vi "Meas Proc QWTB Export Result.vi"(8 "error in":errorcluster, 10 "export data":string[][](array[string]), 11 "qwtb view":T2) -> (0 "error out":errorcluster)   [LabVIEW 2020]
doc: "QWTB result export panel."
uses:
  Meas Proc QWTB Export Mode.ctl
  MEas Proc QWTB Export Sheet Name Mode.ctl
  Meas Proc QWTB Viewer References.ctl
  Meas Proc QWTB View Max Dim.ctl
  Meas Proc QWTB View Uncertainty Mode.ctl
  Meas Proc QWTB View Group Mode.ctl
  Meas Proc QWTB View Phase Mode.ctl
  Meas Proc QWTB Export Sheet Pos.ctl
  varilib/SGUI Assign References Mode.ctl
  Excel/axex_cell_xy.ctl
  GUI/GUI Waveform Info.ctl
  <vilib>/Utility/miscctls.llb/LVRowAndColumnTypeDef.ctl
  Excel/axex_write_cells.vi
  varilib/varilib.lvlib
  Excel/AX Excel.lvlib
panel:
  in  "btn refresh":bool
  in  "sheet pos":T1 caption="New worksheet position"
  in  "trg workbook":u16(ring) caption="Target workbook" items=[">>> No Workbooks <<<"]
  in  "comment":string caption="Comment (Shift+Enter to break line)"
  in  "cb add header":bool caption="Append session header"
  in  "btn cancel":bool
  in  "btn export":bool
  out "sh name prev":string caption="Sheet name preview"
  in  "sh name mode":T3=enum."%Alg Name% %timestamp%" caption="Auto name"
  in  "sh name":string caption="New sheet name"
  in  "exp mode":T4 caption="Export mode"
  out "tbl preview":string[][](table) caption="Preview"
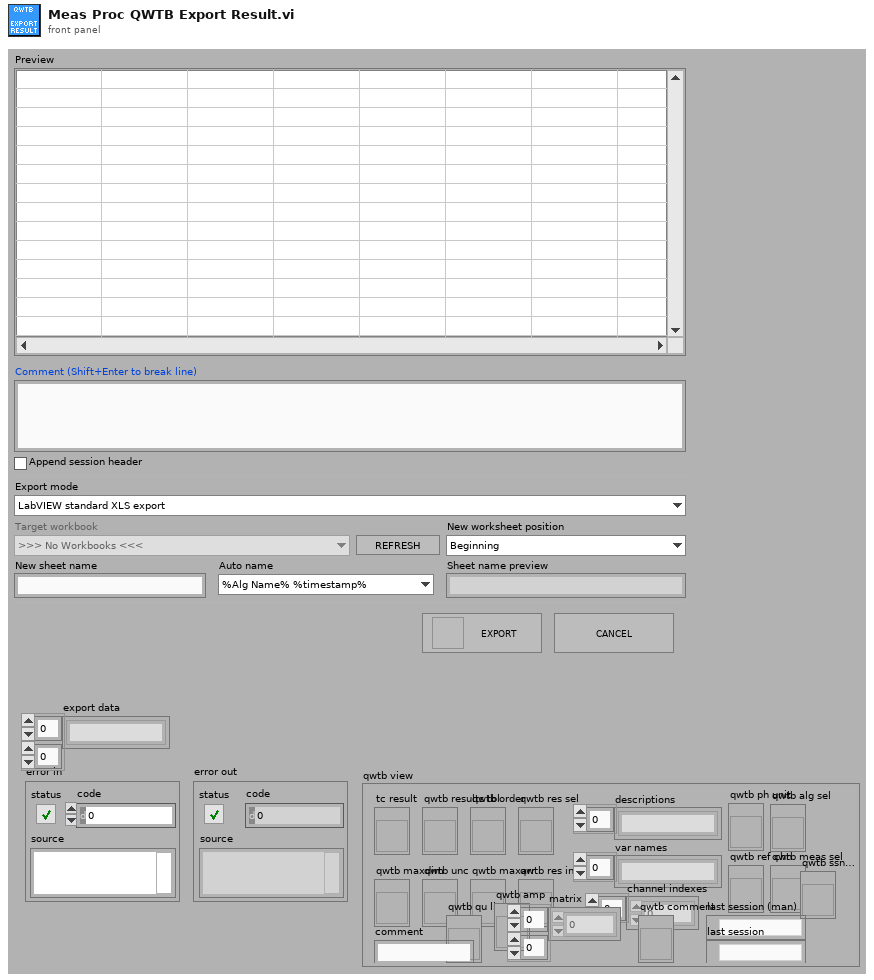
[diagram p1: front panel]
types:
  T1 = typedef "Meas Proc QWTB Export Sheet Pos.ctl" = enum16{"Beginning", "End"}
  T2 = typedef "Meas Proc QWTB Viewer References.ctl" = cluster{"tc result":refnum<vi>, "qwtb results tbl":refnum<vi>, "qwtb maxdim":refnum<vi>, "qwtb unc":refnum<vi>, "qwtb order":refnum<vi>, "qwtb maxarr":refnum<vi>, "qwtb res sel":refnum<vi>, "qwtb res info":refnum<vi>, "descriptions":string[], "var names":string[], "channel indexes":i32[], "qwtb ref chn":refnum<vi>, "qwtb ph unit":refnum<vi>, "qwtb alg sel":refnum<vi>, "qwtb meas sel":refnum<vi>, "qwtb ssn info":refnum<vi>, "last session (man)":path, "qwtb qu list":refnum<vi>, "qwtb amp":refnum<vi>, "matrix":dbl[][], "comment":string, "qwtb comment":refnum<vi>, "last session":path}
  T3 = typedef "MEas Proc QWTB Export Sheet Name Mode.ctl" = enum16{"No", "%Sheet Name% %timestamp%", "%Alg Name% %timestamp%"}
  T4 = typedef "Meas Proc QWTB Export Mode.ctl" = enum16{"LabVIEW standard XLS export", "AX Excel to active workbook", "AX Excel to selected workbook", "AX Excel to new workbook"}
  T5 = typedef "varilib.lvlib/SGUI Assign References Mode.ctl" = enum16{"Add to stack", "Overwrite", "Release last", "Release ID"}
  T6 = typedef "AX Excel.lvlib/axex_cell_xy.ctl" = cluster{"column":i32, "row":i32, "cell name":string}
  T7 = typedef "LVRowAndColumnTypeDef.ctl" = cluster{"Row":i32, "Column":i32}
  T8 = typedef "GUI Waveform Info.ctl" = cluster{"header path":path, "group id":i32, "average id":i32, "Time Stamp":timestamp, "max samples":i64, "first sample":i64, "first smpl [%]":dbl, "kill viewer":bool}
  T9 = typedef "AX Excel.lvlib/axex_instance.ctl" = cluster{"file path":path, "current sheet name":string, "sheet ref":refnum<k7>, "wbook ref":refnum<k7>}
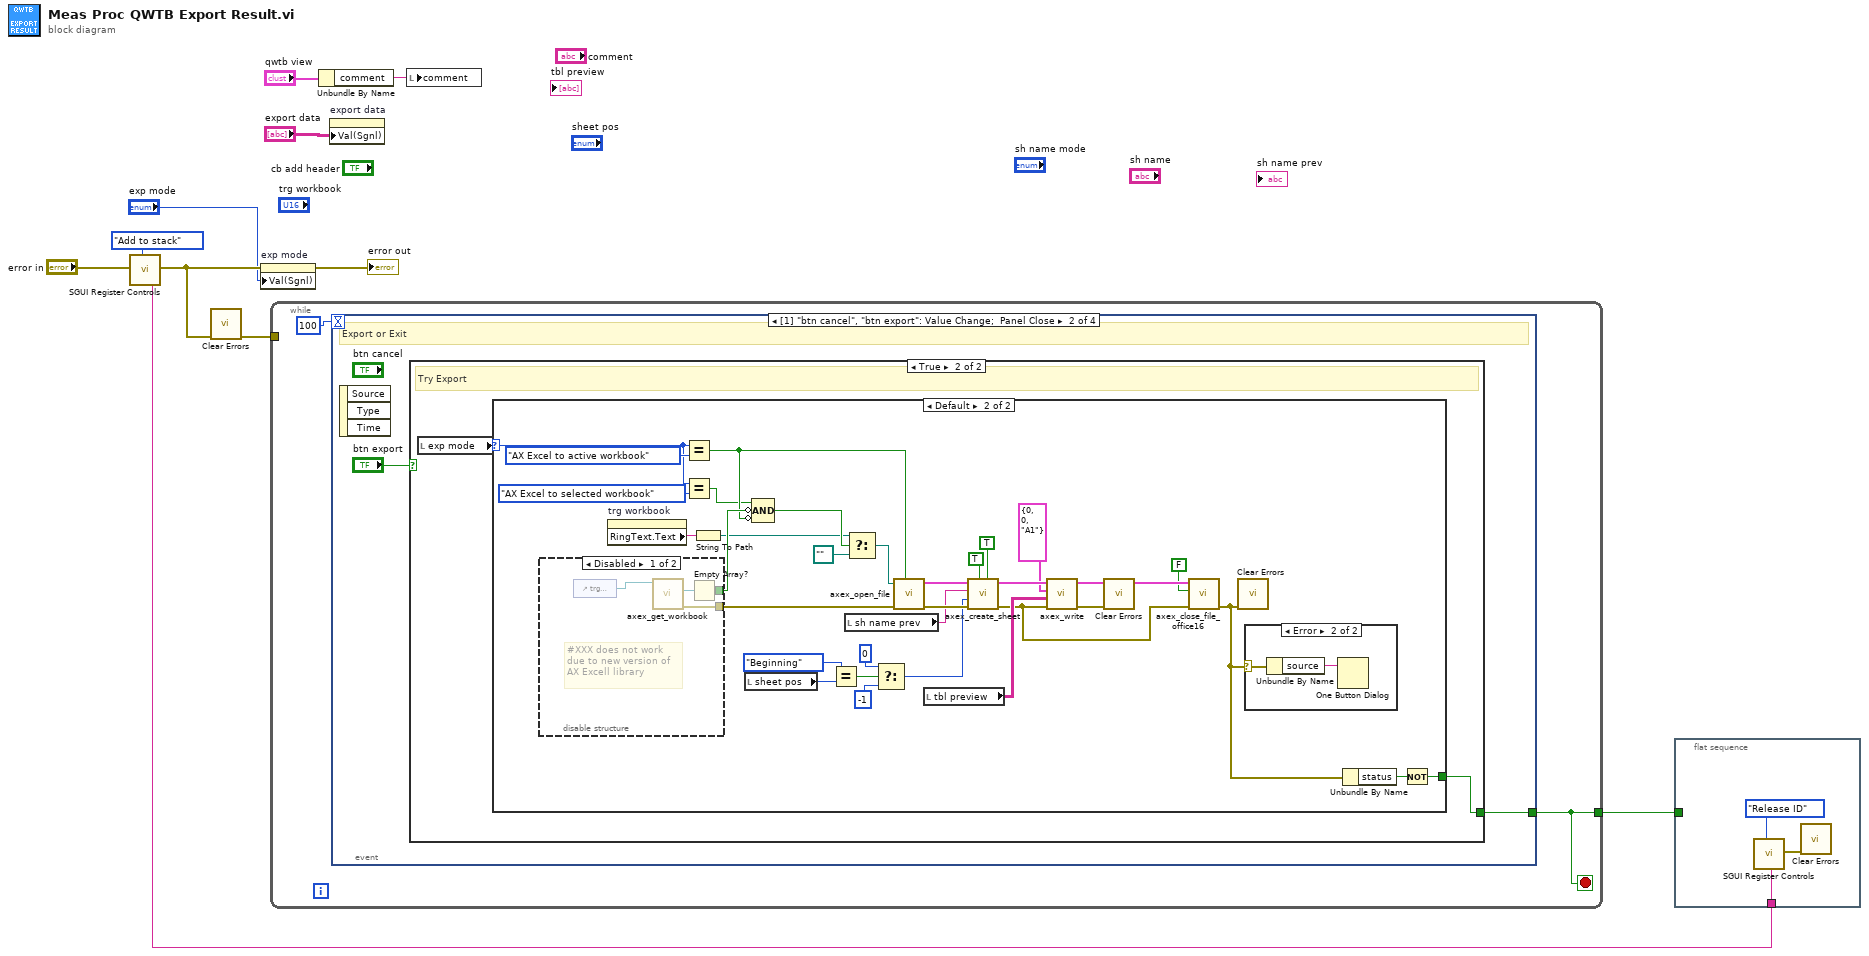
[diagram p0: block diagram]
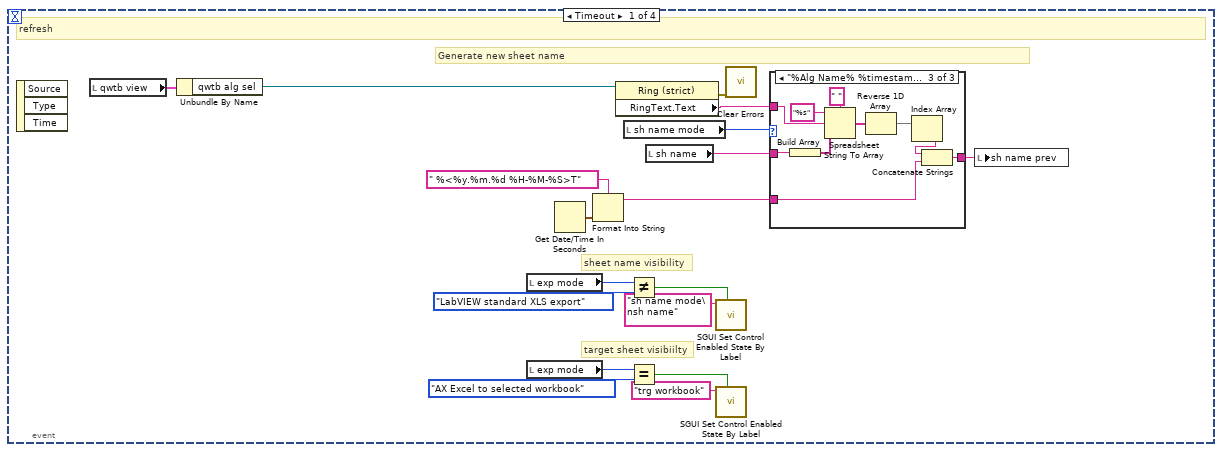
[diagram p2: hidden frame]
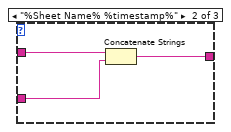
[diagram p4: hidden frame]
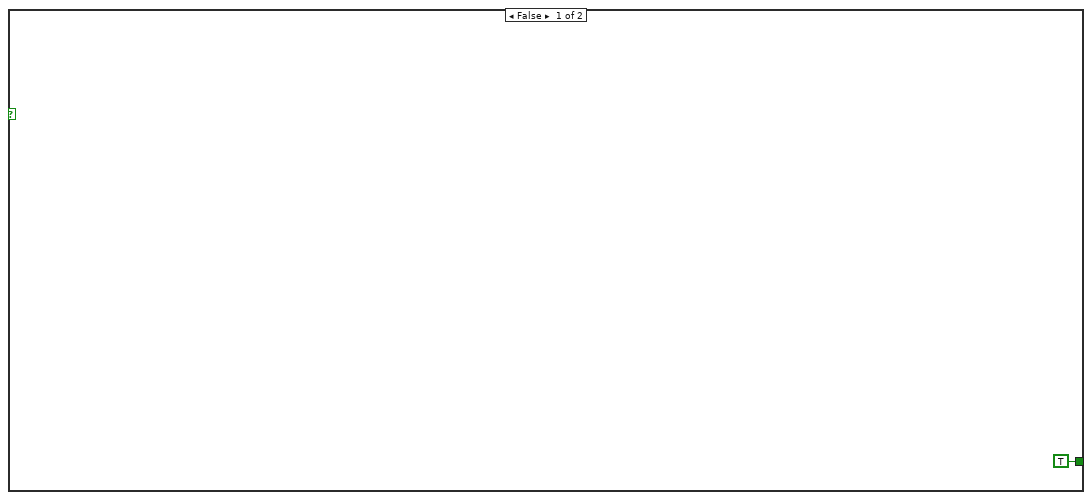
[diagram p5: hidden frame]
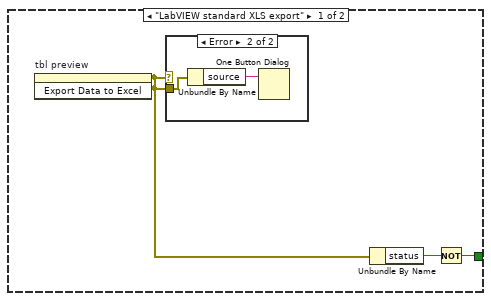
[diagram p6: hidden frame]
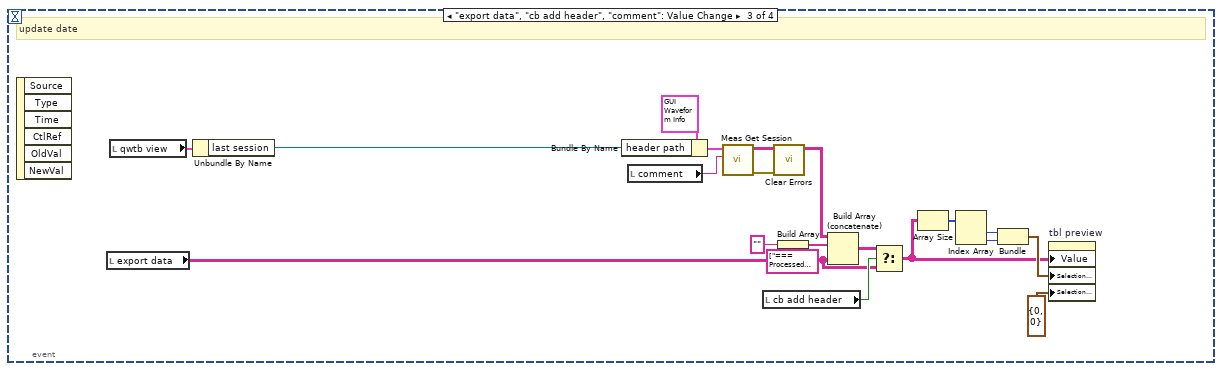
[diagram p10: hidden frame]
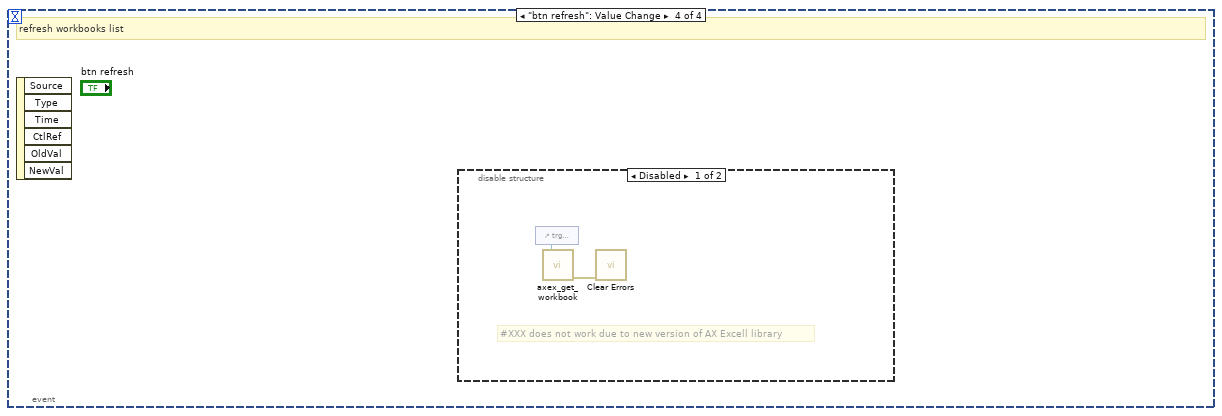
[diagram p11: hidden frame]
diagram:
  n1 = call "SGUI Register Controls.vi"("error in"="error in", "register mode (overwrite)"=SGUI_Assign_References_Mode."Add to stack") -> ("assigned ID"=w8:string, "error out"=w3:errorcluster)  [unwired: 15 in, 1 out]
  n2 = call <vilib>:"Clear Errors.vi"("error in (no error)"=w3) -> ("error out"=w9:errorcluster)  [unwired: 5 in, 1 out]
  n3 = property on="exp mode" class="Enum (strict)"(error in=w3, "Val(Sgnl)"="exp mode") -> (error out=→"error out":errorcluster)  [unwired: 1 in, 1 out]
  n4 = while {
    tunnel: w9 -> [_]
    tunnel: [w13] -> w7
    stop <- w13 stop-if-true
    n5 = event shown="[1] \"btn cancel\", \"btn export\": Value Change;  Panel Close" {
      selector: _ -> [_ _ _ _]
      dyn-events: _ -> [_ _ _ _]
      timeout: 100 -> [_ _ _ _]
      tunnel: [_ w46 _ _] -> w13
      event Timeout {
        # "target sheet visibiilty"
        # "sheet name visibility"
        # "Generate new sheet name"
        # "refresh"
        n6 = event-data() -> ()  [unwired: 1 in, 3 out]
        n7 = local read "qwtb view"() -> (w31:T2)
        n8 = Unbundle By Name(w31) -> ("qwtb alg sel"=w30:refnum<vi>)
        n9 = local read "exp mode"() -> (w22:T4)
        n10 = local read "exp mode"() -> (w14:T4)
        n11 = Get Date/Time In Seconds() -> (seconds since 1Jan1904=w25:timestamp)
        n12 = Format Into String(format string=" %<%y.%m.%d %H-%M-%S>T", w25) -> (resulting string=w24:string)  [unwired: 2 in, 1 out]
        n13 = property class="Ring (strict)"(reference=w30) -> (error out=w18:errorcluster, "RingText.Text"=w27:string)  [unwired: 1 in, 1 out]
        n14 = local read "sh name mode"() -> (w29:T3)
        n15 = Not Equal?(x=w22, y=Meas_Proc_QWTB_Export_Mode."LabVIEW standard XLS export") -> (x != y?=w20:bool)
        n16 = Equal?(x=w14, y=Meas_Proc_QWTB_Export_Mode."AX Excel to selected workbook") -> (x = y?=w16:bool)
        n17 = local read "sh name"() -> (w28:string)
        n18 = call "SGUI Set Control Enabled State By Label.vi"("labels (empty)"="sh name mode\nsh name", "Enabled? (False)"=w20) -> ()  [unwired: 8 in, 2 out]
        n19 = call "SGUI Set Control Enabled State By Label.vi"("labels (empty)"="trg workbook", "Enabled? (False)"=w16) -> ()  [unwired: 8 in, 2 out]
        n20 = call <vilib>:"Clear Errors.vi"("error in (no error)"=w18) -> ()  [unwired: 5 in, 2 out]
        n21 = case shown="\"%Alg Name% %timestamp%\"" w29 {
          tunnel: w28 -> [w32 w35 w40]
          tunnel: w27 -> [_ _ w43]
          tunnel: w24 -> [_ w34 w45]
          tunnel: [w32 w33 w44] -> w23
          frame "No", Default {
          }
          frame "%Sheet Name% %timestamp%" {
            n22 = Concatenate Strings(w35, w34) -> (w33:string)
          }
          frame "%Alg Name% %timestamp%" {
            n23 = Build Array(w40) -> (w39:string[])
            n24 = Spreadsheet String To Array(delimiter (Tab)=" ", format string="%s", spreadsheet string=w43, array type (2D Dbl)=w39) -> (array=w38:string[])
            n25 = Reverse 1D Array(array=w38) -> (reversed array=w37:string[])
            n26 = Index Array(array=w37) -> (element=w36:string)  [unwired: 1 in]
            n27 = Concatenate Strings(w36, w45) -> (w44:string)
          }
        }
        n28 = local write "sh name prev"(w23) -> ()
      }
      event "btn cancel", "btn export": Value Change; Panel Close {
        # "Export or Exit"
        n29 = event-data() -> ()  [unwired: 1 in, 3 out]
        n30 = case shown="True" "btn export" {
          tunnel: [TRUE w49] -> w46
          frame False {
          }
          frame True {
            # "Try Export"
            n31 = local read "exp mode"() -> (w50:T4)
            n32 = case shown="Default" w50 {
              selector: w50 -> [_ w60]
              tunnel: [w52 w76] -> w49
              frame "LabVIEW standard XLS export" {
                n33 = invoke on="tbl preview" class="Tbl (strict)" method="Export Data to Excel"() -> (error out=w51:errorcluster)  [unwired: 3 in, 2 out]
                n34 = case shown="Error" w51 {
                  tunnel: w51 -> [_ w54]
                  frame No Error {
                  }
                  frame Error {
                    n35 = Unbundle By Name(w54) -> ("source"=w55:string)
                    n36 = One Button Dialog(message=w55) -> ()  [unwired: 1 in, 1 out]
                  }
                }
                n37 = Unbundle By Name(w51) -> ("status"=w53:bool)
                n38 = Not(x=w53) -> (.not. x?=w52:bool)
              }
              frame Default {
                n39 = disable-structure shown="Disabled" {
                  disable-tunnel: [w92 _] -> w68
                  disable-tunnel: [w89 _] -> w67
                  frame Disabled {
                    # "#XXX does not work\ndue to new version of\nAX Excell library"
                    n40 = control-ref of="trg workbook"() -> (w91:refnum<vi>)
                    n41 = call "axex_get_workbook.vi"("AX Excel instance in"=w91) -> ("error out"=w92:errorcluster, "excel workbook"=w90:refnum<k7>)  [unwired: 8 in, 1 out]
                    n42 = Empty Array?(array=w90) -> (empty?=w89:bool)
                  }
                  frame Enabled {
                  }
                }
                n43 = property on="trg workbook" class="Ring (strict)"() -> ("RingText.Text"=w75:string)  [unwired: 2 in, 2 out]
                n44 = Equal?(x=w60, y=Meas_Proc_QWTB_Export_Mode."AX Excel to active workbook") -> (x = y?=w65:bool)
                n45 = Equal?(x=w60, y=Meas_Proc_QWTB_Export_Mode."AX Excel to selected workbook") -> (x = y?=w61:bool)
                n46 = String To Path(string=w75) -> (path=w63:path)
                n47 = local read "sheet pos"() -> (w74:T1)
                n48 = Compound Arithmetic op=AND(w61, invert w67, invert w65) -> (w64:bool)
                n49 = Equal?(x=Meas_Proc_QWTB_Export_Sheet_Pos."Beginning", y=w74) -> (x = y?=w73:bool)
                n50 = local read "sh name prev"() -> (w84:string)
                n51 = Select(t=w63, s=w64, f=path "" ("t")) -> (s? t:f=w66:path)
                n52 = Select(t=0, s=w73, f=-1) -> (s? t:f=w69:i32)
                n53 = call "axex_open_file.vi"("open active workbook (False)"=w65, "error in"=w68, "excel file path (full)"=w66) -> ("error out"=w88:errorcluster, "AX Excel instance out"=w87:T9)  [unwired: 7 in]
                n54 = local read "tbl preview"() -> (w78:string[][])
                n55 = call "axex_create_sheet.vi"("activate sheet (False)"=TRUE, "select new sheet (False)"=TRUE, "error in"=w88, "position index (-1: last)"=w69, "new sheet name"=w84, "AX Excel instance in"=w87) -> ("error out"=w56:errorcluster, "AX Excel instance out"=w83:T9)  [unwired: 4 in]
                n56 = call-poly "axex_write.vi"("error in"=w56, "cell array"=w78, "top left cell"=T6 {"column"=0, "row"=0, "cell name"="A1"}, "AX Excel instance in"=w83) -> ("error out"=w57:errorcluster, "AX Excel instance out"=w82:T9)  [unwired: 6 in]
                n57 = call <vilib>:"Clear Errors.vi"("error in (no error)"=w57) -> ()  [unwired: 5 in, 2 out]
                n58 = call "axex_close_file_office16.vi"("error in"=w56, "save changes (True)"=FALSE, "AX Excel instance in"=w82) -> ("error out"=w58:errorcluster)  [unwired: 8 in]
                n59 = call <vilib>:"Clear Errors.vi"("error in (no error)"=w58) -> ()  [unwired: 5 in, 2 out]
                n60 = case shown="Error" w58 {
                  selector: w58 -> [_ w93]
                  frame No Error {
                  }
                  frame Error {
                    n61 = Unbundle By Name(w93) -> ("source"=w94:string)
                    n62 = One Button Dialog(message=w94) -> ()  [unwired: 1 in, 1 out]
                  }
                }
                n63 = Unbundle By Name(w58) -> ("status"=w79:bool)
                n64 = Not(x=w79) -> (.not. x?=w76:bool)
              }
            }
          }
        }
      }
      event "export data", "cb add header", "comment": Value Change {
        # "update date"
        n65 = event-data() -> ()  [unwired: 1 in, 6 out]
        n66 = local read "export data"() -> (w106:string[][])
        n67 = local read "qwtb view"() -> (w113:T2)
        n68 = Unbundle By Name(w113) -> ("last session"=w111:path)
        n69 = Bundle By Name(cluster=T8 {"header path"=path "", "group id"=1, "average id"=0, "Time Stamp"=timestamp(0 s since 1904-01-01), "max samples"=0, "first sample"=0, "first smpl [%]"=-1.0, "kill viewer"=FALSE} ("record info"), "header path"=w111) -> (w110:T8)
        n70 = local read "comment"() -> (w105:string)
        n71 = call "Meas Get Session.vi"("comment override"=w105, "record info"=w110) -> ("error out"=w109:errorcluster, "config matrix"=w98:string[][])  [unwired: 8 in]
        n72 = local read "cb add header"() -> (w108:bool)
        n73 = call <vilib>:"Clear Errors.vi"("error in (no error)"=w109) -> ()  [unwired: 5 in, 2 out]
        n74 = Build Array("") -> (w96:string[])
        n75 = Build Array (concatenate)(w98, w96, string[] ["=== Processed Data ==="] ("element"), w106) -> (w107:string[][])
        n76 = Select(t=w107, s=w108, f=w106) -> (s? t:f=w102:string[][])
        n77 = Array Size(array=w102) -> (size(s)=w101:i32[])
        n78 = Index Array(array=w101) -> (element #1=w100:i32, element #2=w99:i32)  [unwired: 2 in]
        n79 = Bundle(w100, w99) -> (w103:cluster{i32, i32})  [unwired: 1 in]
        n80 = property on="tbl preview" class="Tbl (strict)"("Value"=w102, "Selection Size"=w103, "Selection Start"=T7 {"Row"=0, "Column"=0} ("Selection Size")) -> ()  [unwired: 2 in, 2 out]
      }
      event "btn refresh": Value Change {
        # "refresh workbooks list"
        n81 = event-data() -> ()  [unwired: 1 in, 6 out]
        n82 = disable-structure shown="Disabled" {
          frame Disabled {
            # "#XXX does not work due to new version of AX Excell library"
            n83 = control-ref of="trg workbook"() -> (w115:refnum<vi>)
            n84 = call "axex_get_workbook.vi"("AX Excel instance in"=w115) -> ("error out"=w114:errorcluster)  [unwired: 8 in, 2 out]
            n85 = call <vilib>:"Clear Errors.vi"("error in (no error)"=w114) -> ()  [unwired: 5 in, 2 out]
          }
          frame Enabled {
          }
        }
      }
    }
  }
  n86 = Unbundle By Name("qwtb view") -> ("comment"=w4:string)
  n87 = property on="export data" class="Arr (strict)"("Val(Sgnl)"="export data") -> ()  [unwired: 2 in, 2 out]
  n88 = local write "comment"(w4) -> ()
  n89 = flat-sequence {
    tunnel: w8 -> [w117]
    tunnel: w7 -> [_]
    frame #0 {
      n90 = call "SGUI Register Controls.vi"("register mode (overwrite)"=SGUI_Assign_References_Mode."Release ID", "controls ID (empty)"=w117) -> ("error out"=w116:errorcluster)  [unwired: 15 in, 2 out]
      n91 = call <vilib>:"Clear Errors.vi"("error in (no error)"=w116) -> ()  [unwired: 5 in, 2 out]
    }
  }
